vi "Core Action.vi"(8 "error in (no error)":errorcluster, 10 "SECS-II Class":refnum<class "SECS-II Class.lvclass">, 11 "11-Alarm Management in":refnum<class "11-Alarm Management.lvclass">) -> (0 "error out":errorcluster, 2 "SECS-II Class Out":refnum<class "SECS-II Class.lvclass">, 3 "11-Alarm Management out":refnum<class "11-Alarm Management.lvclass">)   [LabVIEW 2020, in "SECS Scenarios.lvlib" / "11-Alarm Management.lvclass"]
uses:
  11-Alarm Management.lvclass
  D:/Dropbox/SECS/SECS_GEM v1.1.0/Com/SECS Scenarios/Scenarios Class/Scenarios Class.lvclass
  SECS Communication/SECS-II Class/SECS-II Class.lvclass
  11-Alarm Management.lvclass/11-Alarm Management.ctl
  SECS Communication/S5 Message Class/S5F1.ctl
  SECS Communication/S5 Message Class/S5 Message Class.lvclass
  D:/Dropbox/SECS/SECS_GEM v1.1.0/Com/SECS Communication/SECS-II Class/SECS-II Class.lvclass
  Scenarios Class/Scenarios Class.lvclass/Scenarios Class.ctl
  Scenarios Class/Reply State.ctl
  Scenarios Class/Write Reply State.vi
  Scenarios Class/Read HSMS Class.vi
  SECS Communication/SECS Data Class/Get ALID Data.vi
  SECS Communication/HSMS Class/HSMS Class.lvclass
  SECS Communication/SECS Data Class/SECS Data Class.lvclass
  Scenarios Class/Scenarios Class.lvclass
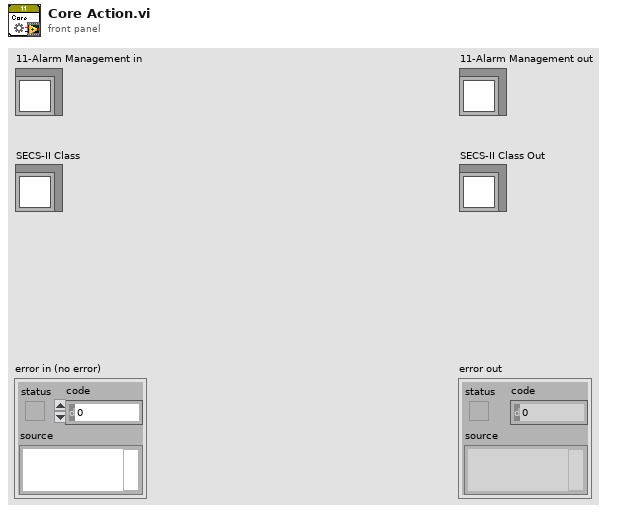
[diagram p1: front panel]
types:
  T1 = typedef "SECS Communication.lvlib/SECS Data Class.lvclass/ALID Data.ctl" = cluster{"Enable":bool, "ALID":u32, "Name":string, "Description":string, "Source":string, "Status":enum16{"Null", "Normal", "Abnormal", "Warning"}}
  T2 = typedef "SECS Communication.lvlib/S5 Message Class.lvclass/S5F1.ctl" = cluster{"ALCD(Bit8)":bool, "ALID":u32, "ALTX":string}
  T3 = typedef "SECS Scenarios.lvlib/Scenarios Class.lvclass/Reply State.ctl" = enum16{"OK", "Illegal Data", "Unknown Stream", "Unknown Function", "Off-Line", "T3 Timeout", "Inner-Timeout"}
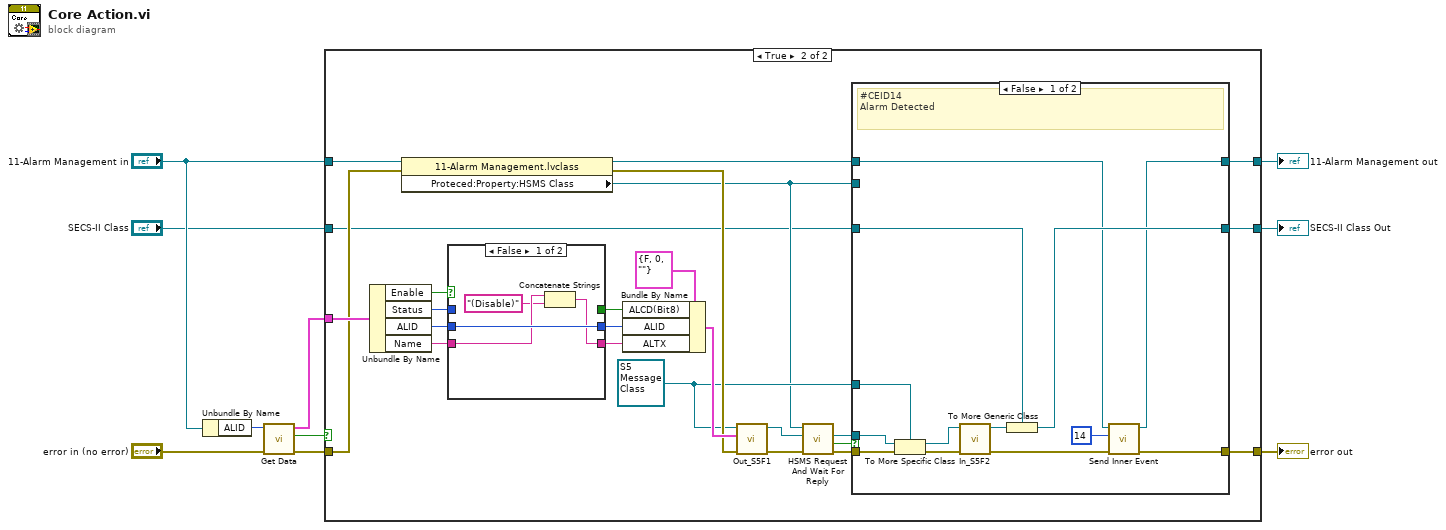
[diagram p0: block diagram]
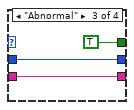
[diagram p5: hidden frame]
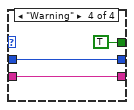
[diagram p6: hidden frame]
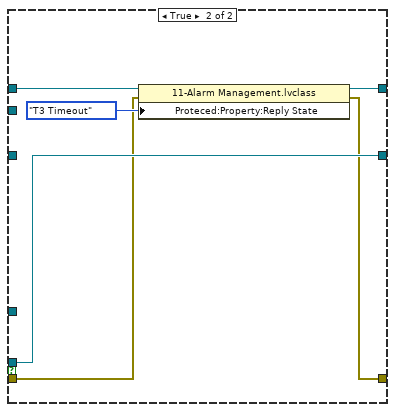
[diagram p7: hidden frame]
diagram:
  n1 = Unbundle By Name("11-Alarm Management in") -> ("ALID"=w9:u32)
  n2 = call-poly "Get Data.vi"("error in"="error in (no error)", "ALID"=w9) -> ("error out"=w7:errorcluster, "Find?"=w6:bool, "ALID Data"=w8:T1)  [unwired: 7 in]
  n3 = case shown="True" w6 {
    tunnel: w8 -> [_ w38]
    tunnel: w7 -> [w12 w33]
    tunnel: "11-Alarm Management in" -> [w13 w34]
    tunnel: [w13 w23] -> w4
    tunnel: [w12 w26] -> w3
    tunnel: "SECS-II Class" -> [w11 w22]
    tunnel: [w11 w21] -> w1
    frame False {
    }
    frame True {
      w28 = refnum<class "S5 Message Class.lvclass"> refnum ("S5 Message Class in")
      n4 = Unbundle By Name(w38) -> ("Enable"=w20:bool, "Status"=w19:enum16{"Null", "Normal", "Abnormal", "Warning"}, "ALID"=w18:u32, "Name"=w17:string)
      n5 = property class="11-Alarm Management.lvclass"(reference=w34, error in=w33) -> (reference out=w24:refnum<class "11-Alarm Management.lvclass">, error out=w32:errorcluster, "Proteced:Property:HSMS Class"=w27:refnum<class "HSMS Class.lvclass">)
      n6 = case shown="False" w20 {
        tunnel: w19 -> [_ w48]
        tunnel: w18 -> [w42 w47]
        tunnel: w17 -> [w41 w46]
        tunnel: [w40 w45] -> w16
        tunnel: [w42 w44] -> w15
        tunnel: [_ w43] -> w14
        frame False {
          n7 = Concatenate Strings(w41, "(Disable)" ("string")) -> (w40:string)
        }
        frame True {
          n8 = case shown="\"Normal\"" w48 {
            tunnel: w47 -> [w50 w51 w54 w57]
            tunnel: w46 -> [w49 w52 w55 w58]
            tunnel: [w49 w52 w55 w58] -> w45
            tunnel: [w50 w51 w54 w57] -> w44
            tunnel: [_ _ TRUE TRUE] -> w43
            frame "Null", Default {
            }
            frame "Normal" {
            }
            frame "Abnormal" {
            }
            frame "Warning" {
            }
          }
        }
      }
      n9 = Bundle By Name(cluster=T2 {"ALCD(Bit8)"=FALSE, "ALID"=0, "ALTX"=""} ("S5F1"), "ALCD(Bit8)"=w14, "ALID"=w15, "ALTX"=w16) -> (w36:T2)
      n10 = call "Out_S5F1.vi"("error in (no error)"=w32, "S5F1"=w36, "S5 Message Class in"=w28) -> ("error out"=w31:errorcluster, "S5 Message Class out"=w35:refnum<class "S5 Message Class.lvclass">)  [unwired: 7 in]
      n11 = call "HSMS Request And Wait For Reply.vi"("error in (no error)"=w31, "SECS-II Class In"=w35, "HSMS Class in"=w27) -> ("error out"=w30:errorcluster, "Timeout?"=w25:bool, "SECS-II Class Out"=w29:refnum<class "SECS-II Class.lvclass">)  [unwired: 5 in, 1 out]
      n12 = case shown="False" w25 {
        tunnel: w30 -> [w71 w73]
        tunnel: w29 -> [w70 w77]
        tunnel: w28 -> [w69 _]
        tunnel: w27 -> [_ _]
        tunnel: [w60 w72] -> w26
        tunnel: w24 -> [w62 w76]
        tunnel: [w61 w74] -> w23
        tunnel: w22 -> [w65 _]
        tunnel: [w64 w77] -> w21
        frame False {
          # "#CEID14\nAlarm Detected"
          n13 = To More Specific Class(target class=w69, reference=w70, error in=w71) -> (specific class reference=w67:refnum<class "S5 Message Class.lvclass">, error out=w68:errorcluster)
          n14 = call "In_S5F2.vi"("error in (no error)"=w68, "S5 Message Class in"=w67) -> ("error out"=w63:errorcluster, "S5 Message Class out"=w66:refnum<class "S5 Message Class.lvclass">)  [unwired: 6 in, 2 out]
          n15 = To More Generic Class(target class=w65, reference=w66) -> (generic class reference=w64:refnum<class "SECS-II Class.lvclass">)
          n16 = call "Send Inner Event.vi"("error in (no error)"=w63, "CEID"=u32 14, "Scenarios Class in"=w62) -> ("error out"=w60:errorcluster, "Scenarios Class out"=w61:refnum<class "11-Alarm Management.lvclass">)  [unwired: 7 in]
        }
        frame True {
          n17 = property class="11-Alarm Management.lvclass"(reference=w76, error in=w73, "Proteced:Property:Reply State"=Reply_State."T3 Timeout" ("Reply State")) -> (reference out=w74:refnum<class "11-Alarm Management.lvclass">, error out=w72:errorcluster)
        }
      }
    }
  }
  "error out" <- w3
  "11-Alarm Management out" <- w4
  "SECS-II Class Out" <- w1
